vi "applyNewForceDemand.vi"(8 "error in (no error)":errorcluster, 10 "Force Demand":T1 format="%.6f", 11 "Model in":refnum<class "Model.lvclass">) -> (0 "error out":errorcluster, 3 "Model out":refnum<class "Model.lvclass">)   [LabVIEW 2013, in "Model.lvclass"]
uses:
  Model.lvclass
  Typedefs/ForceDemand.ctl
  Model.lvclass/Model.ctl
  ApplicationElements/SystemController/SystemController.lvclass/SystemController.ctl
  ApplicationElements/SystemController/SystemController.lvclass
  Typedefs/M2AADTTypedefs.lvlib
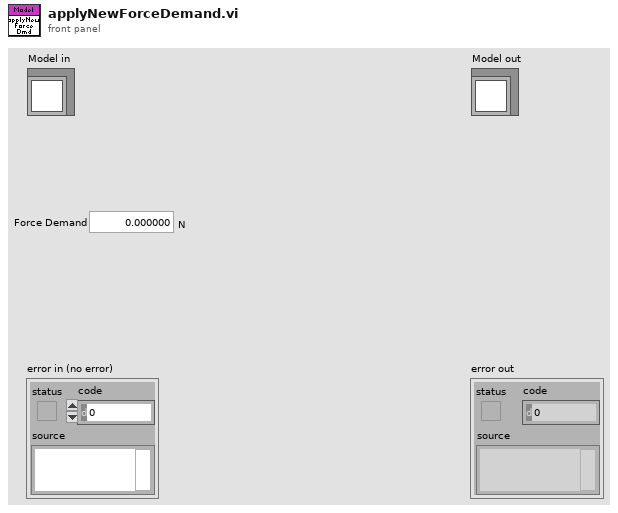
[diagram p1: front panel]
types:
  T1 = typedef "M2AADTTypedefs.lvlib/ForceDemand.ctl" = dbl[unit]
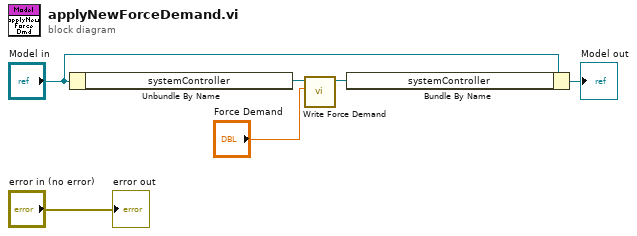
[diagram p0: block diagram]
diagram:
  n1 = Unbundle By Name("Model in") -> ("systemController"=w5:refnum<class "SystemController.lvclass">)
  n2 = call "Write Force Demand.vi"("Force Demand"="Force Demand", "SystemController in"=w5) -> ("SystemController out"=w1:refnum<class "SystemController.lvclass">)  [unwired: 9 in]
  n3 = Bundle By Name(cluster="Model in", "systemController"=w1) -> (→"Model out":refnum<class "Model.lvclass">)
  "error out" <- "error in (no error)"
